vi "ChangeMethodTreeSelection.vi"(7 "TreeControl in":refnum<vi>, 8 "Interfaces":string[](array[string]), 9 "MethodsPerInterfaces":cluster{"Array":string[]}[](array[cluster]), 10 "MouseClickCoordinates":T1, 11 "SelectedMethodsIn":cluster{"Array":bool[]}[](array[cluster])) -> (3 "SelectedMethodsOut":cluster{"Array":bool[]}[](array[cluster]))   [LabVIEW 2020, in "InterfaceLibrary.lvlib"]
uses:
  InterfaceLibrary.lvlib
  <vilib>/Utility/miscctls.llb/LVPoint32TypeDef.ctl
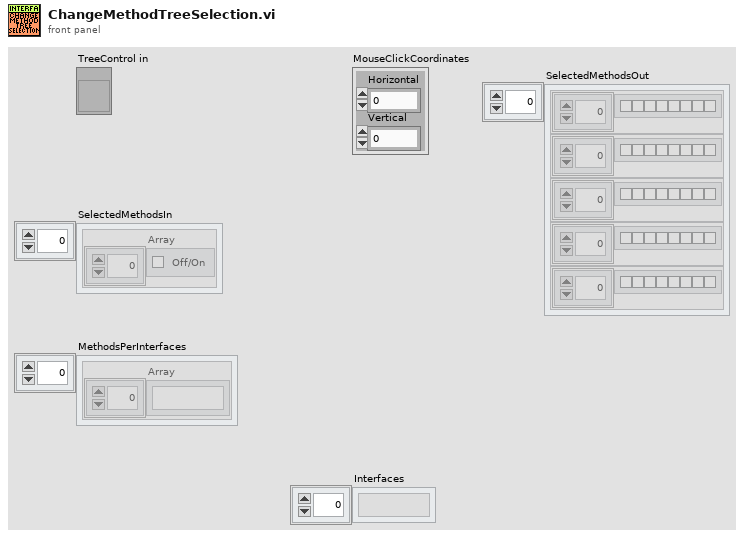
[diagram p1: front panel]
types:
  T1 = typedef "LVPoint32TypeDef.ctl" = cluster{"Horizontal":i32, "Vertical":i32}
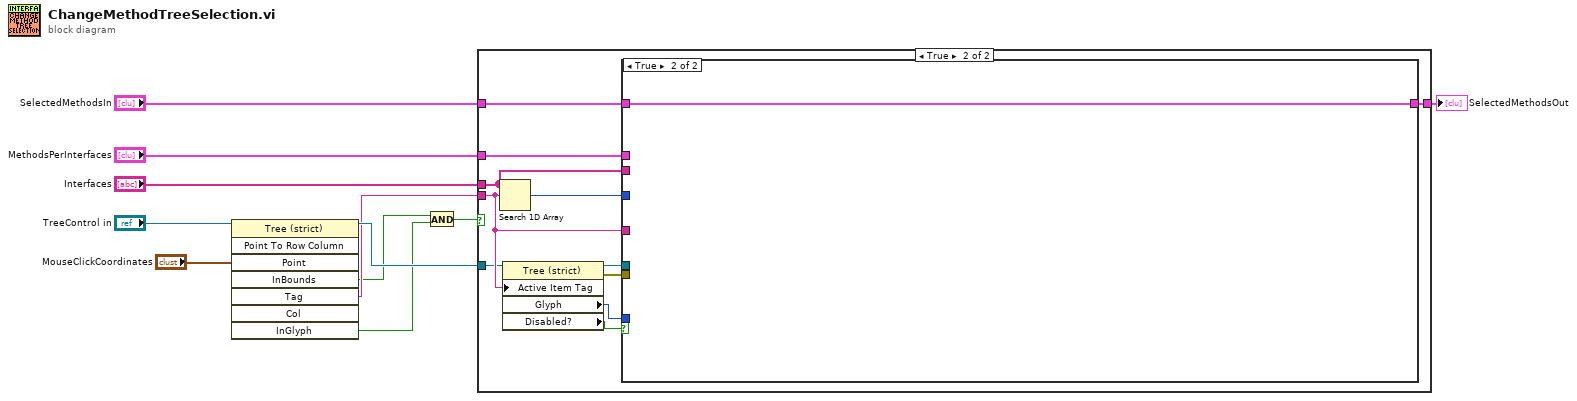
[diagram p0: block diagram]
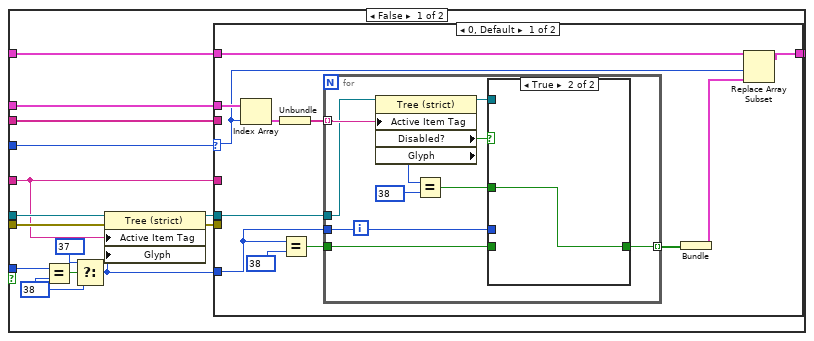
[diagram p3: hidden frame]
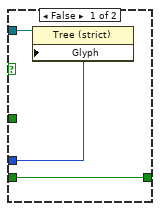
[diagram p4: hidden frame]
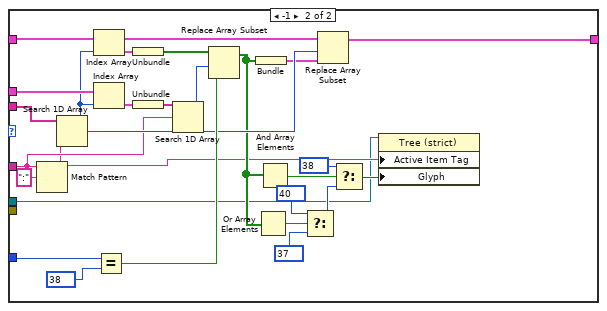
[diagram p5: hidden frame]
diagram:
  n1 = invoke on="Invoke Node" class="Tree (strict)" method="Point To Row Column"(reference="TreeControl in", "Point"="MouseClickCoordinates") -> (reference out=w11:refnum<vi>, "InBounds"=w2:bool, "Tag"=w6:string, "InGlyph"=w3:bool)  [unwired: 6 in, 4 out]
  n2 = And(x=w2, y=w3) -> (x .and. y?=w4:bool)
  n3 = case shown="True" w4 {
    tunnel: "Interfaces" -> [_ w22]
    tunnel: w6 -> [_ w16]
    tunnel: "MethodsPerInterfaces" -> [_ w21]
    tunnel: "SelectedMethodsIn" -> [w12 w18]
    tunnel: [w12 w17] -> w8
    tunnel: w11 -> [_ w15]
    frame False {
    }
    frame True {
      n4 = Search 1D Array(1D array=w22, element=w16) -> (index of element=w23:i32)  [unwired: 1 in]
      n5 = property on="Property Node" class="Tree (strict)"(reference=w15, "Active Item Tag"=w16) -> (reference out=w14:refnum<vi>, error out=w20:errorcluster, "Glyph"=w19:i32, "Disabled?"=w13:bool)  [unwired: 1 in]
      n6 = case shown="True" w13 {
        tunnel: w23 -> [w38 _]
        tunnel: w22 -> [w37 _]
        tunnel: w21 -> [w36 _]
        tunnel: w20 -> [w35 _]
        tunnel: w19 -> [w34 _]
        tunnel: w18 -> [w29 w91]
        tunnel: [w28 w91] -> w17
        tunnel: w16 -> [w24 _]
        tunnel: w14 -> [w27 _]
        frame False {
          w25 = 38
          n7 = Equal?(x=w34, y=w25) -> (x = y?=w33:bool)
          n8 = Select(t=37, s=w33, f=w25) -> (s? t:f=w30:i32)
          n9 = property on="Property Node" class="Tree (strict)"(reference=w27, error in=w35, "Active Item Tag"=w24, "Glyph"=w30) -> (reference out=w26:refnum<vi>, error out=w31:errorcluster)
          n10 = case shown="0, Default" w38 {
            selector: w38 -> [w46 _]
            tunnel: w24 -> [_ w67]
            tunnel: w37 -> [_ w89]
            tunnel: w36 -> [w49 w88]
            tunnel: w31 -> [_ _]
            tunnel: w30 -> [w45 w81]
            tunnel: w29 -> [w47 w79]
            tunnel: [w43 w76] -> w28
            tunnel: w26 -> [w39 w65]
            frame 0, Default {
              n11 = Index Array(array=w49, index=w46) -> (element=w50:cluster{"Array":string[]})
              n12 = Unbundle(w50) -> ("Array"=w48:string[])
              n13 = Equal?(x=w45, y=38) -> (x = y?=w41:bool)
              n14 = for {
                tunnel: w48 -> [w60] mode=indexing
                tunnel: w45 -> [w54]
                tunnel: w41 -> [w53]
                tunnel: [w52] -> w40 mode=indexing
                tunnel: w39 -> [w59]
                n15 = property on="Property Node" class="Tree (strict)"(reference=w59, "Active Item Tag"=w60) -> (reference out=w58:refnum<vi>, "Disabled?"=w55:bool, "Glyph"=w57:i32)  [unwired: 1 in, 1 out]
                n16 = Equal?(x=w57, y=38) -> (x = y?=w51:bool)
                n17 = case shown="True" w55 {
                  tunnel: w58 -> [w63 _]
                  tunnel: w54 -> [w61 _]
                  tunnel: w53 -> [w62 _]
                  tunnel: [w62 w64] -> w52
                  tunnel: w51 -> [_ w64]
                  frame False {
                    n18 = property on="Property Node" class="Tree (strict)"(reference=w63, "Glyph"=w61) -> ()  [unwired: 1 in, 2 out]
                  }
                  frame True {
                  }
                }
              }
              n19 = Bundle(w40) -> (w44:cluster{bool[]})  [unwired: 1 in]
              n20 = Replace Array Subset(array=w47, new element=w44, index=w46) -> (w43:cluster{"Array":bool[]}[])
            }
            frame -1 {
              n21 = Match Pattern(string=w67, regular expression=":") -> (before substring=w66:string)  [unwired: 1 in, 3 out]
              n22 = Search 1D Array(1D array=w89, element=w66) -> (index of element=w78:i32)  [unwired: 1 in]
              n23 = Index Array(array=w79, index=w78) -> (element=w85:cluster{"Array":bool[]})
              n24 = Index Array(array=w88, index=w78) -> (element=w87:cluster{"Array":string[]})
              n25 = Equal?(x=w81, y=38) -> (x = y?=w80:bool)
              n26 = Unbundle(w85) -> ("Array"=w84:bool[])
              n27 = Unbundle(w87) -> ("Array"=w86:string[])
              n28 = Search 1D Array(1D array=w86, element=w67) -> (index of element=w83:i32)  [unwired: 1 in]
              n29 = Replace Array Subset(array=w84, new element=w80, index=w83) -> (w75:bool[])
              n30 = Bundle("Array"=w75) -> (w77:cluster{"Array":bool[]})  [unwired: 1 in]
              n31 = Or Array Elements(Boolean array=w75) -> (logical OR=w72:bool)
              n32 = And Array Elements(Boolean array=w75) -> (logical AND=w74:bool)
              n33 = Select(t=40, s=w72, f=37) -> (s? t:f=w71:i32)
              n34 = Replace Array Subset(array=w79, new element=w77, index=w78) -> (w76:cluster{"Array":bool[]}[])
              n35 = Select(t=38, s=w74, f=w71) -> (s? t:f=w68:i32)
              n36 = property on="Property Node" class="Tree (strict)"(reference=w65, "Active Item Tag"=w66, "Glyph"=w68) -> ()  [unwired: 1 in, 2 out]
            }
          }
        }
        frame True {
        }
      }
    }
  }
  "SelectedMethodsOut" <- w8
